vi "Command_MoveArmsToSafety.vi"(7 "Parameters":dbl[](array[numeric]), 11 "Startup":bool) -> (4 "Completed":bool, 6 "Outer_Arm_Pneumatic":T2, 10 "Inner_Arm_Pneumatic":T1, 15 "Reinit":bool)   [LabVIEW 2020]
uses:
  Auto Utilities/Command_Execution_State.ctl
  Subsystems/Climber/Climber_Outer_Arm_Enum.ctl
  Subsystems/Climber/Climber_Inner_Arm_Enum.ctl
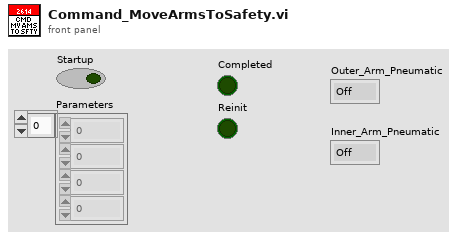
[diagram p1: front panel]
types:
  T1 = typedef "Climber_Inner_Arm_Enum.ctl" = enum16{"Off", "On", "Forward", "Back"}
  T2 = typedef "Climber_Outer_Arm_Enum.ctl" = enum16{"Off", "On", "Vertical", "Back"}
  T3 = typedef "Command_Execution_State.ctl" = enum16{"Initialize", "Execute", "Finish"}
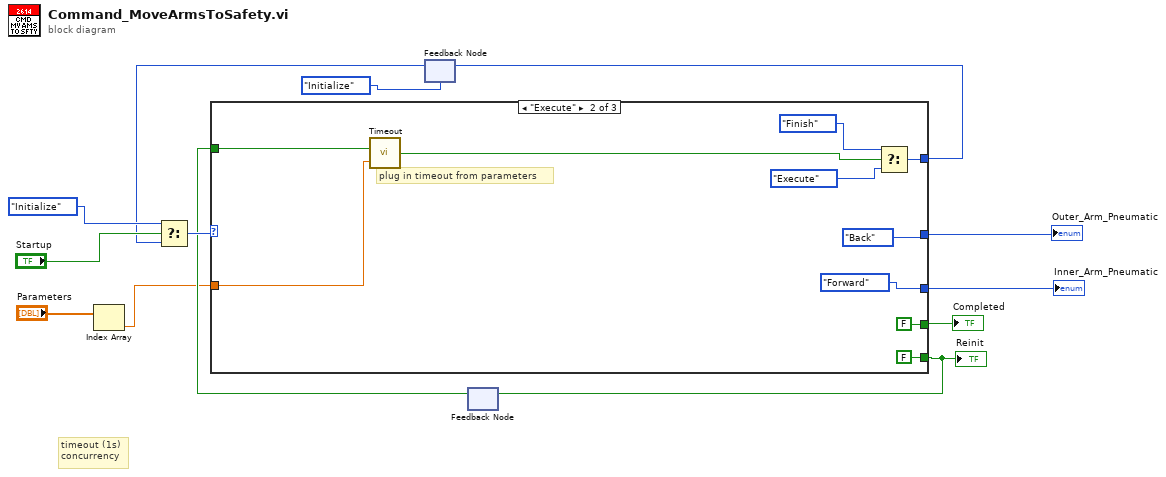
[diagram p0: block diagram]
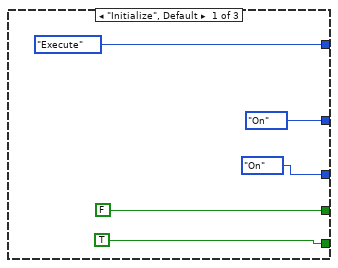
[diagram p2: hidden frame]
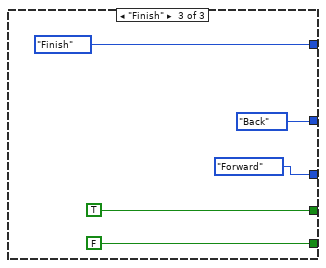
[diagram p3: hidden frame]
diagram:
  # "timeout (1s)\nconcurrency"
  n1 = Index Array(array="Parameters") -> (element=w3:dbl)  [unwired: 1 in]
  n2 = feedback #1(Command_Execution_State."Initialize") -> (w9:T3)
  n3 = Select(t=Command_Execution_State."Initialize", s="Startup", f=w9) -> (s? t:f=w11:T3)
  n4 = feedback #2() -> (w5:bool)  [unwired: 1 in]
  n5 = case shown="\"Execute\"" w11 {
    tunnel: [Command_Execution_State."Execute" w26 Command_Execution_State."Finish"] -> w10
    tunnel: [FALSE ("Reinit") FALSE ("Reinit") TRUE ("Reinit")] -> w7
    tunnel: [TRUE ("Reinit") FALSE ("Reinit") FALSE ("Reinit")] -> w6
    tunnel: w5 -> [_ w23 _]
    tunnel: w3 -> [_ w19 _]
    tunnel: [Climber_Outer_Arm_Enum."On" ("Outer_Arm_Pneumatic") Climber_Outer_Arm_Enum."Back" ("Outer_Arm_Pneumatic") Climber_Outer_Arm_Enum."Back" ("Outer_Arm_Pneumatic")] -> w2
    tunnel: [Climber_Inner_Arm_Enum."On" ("Inner_Arm_Pneumatic") Climber_Inner_Arm_Enum."Forward" ("Inner_Arm_Pneumatic") Climber_Inner_Arm_Enum."Forward" ("Inner_Arm_Pneumatic")] -> w1
    frame "Initialize", Default {
    }
    frame "Execute" {
      # "plug in timeout from parameters"
      n6 = call "Timeout.vi"("Timeout"=w19, "Initialize"=w23) -> ("Timed Out?"=w22:bool)
      n7 = Select(t=Command_Execution_State."Finish", s=w22, f=Command_Execution_State."Execute") -> (s? t:f=w26:T3)
    }
    frame "Finish" {
    }
  }
  "Reinit" <- w6
  "Completed" <- w7
  "Outer_Arm_Pneumatic" <- w2
  "Inner_Arm_Pneumatic" <- w1
  n8 = feedback-in #1(w10) -> ()
  n9 = feedback-in #2(w6) -> ()
